vi "Load WAV.vi"(8 "error in (no error)":errorcluster, 11 "Path":path) -> (0 "error out":errorcluster, 1 "data":waveform(i16)[](array[waveform]), 2 "Sample Rate (Hz)":i32, 3 "Channels":i32, 5 "Length (Samples)":i32)   [LabVIEW 2018, in "Audio File Input.lvlib"]
doc: "Loads a WAV file from disk.\n\n<b>Priority:</b> Background priority (lowest)"
uses:
  Audio File Input.lvlib
  <vilib>/sound2/lvsound2.llb/Sound File Read Open.vi
  <vilib>/sound2/lvsound2.llb/Sound File Info (refnum).vi
  <vilib>/sound2/lvsound2.llb/Sound File Read (I16).vi
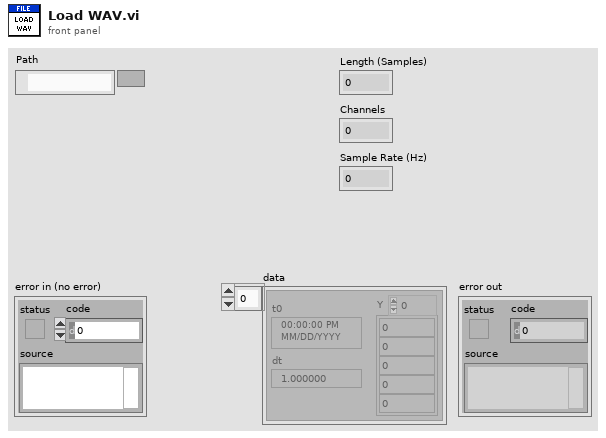
[diagram p1: front panel]
types:
  T1 = typedef "Sound File Refnum.ctl" = refnum<file>
  T2 = typedef "Sound Data Format.ctl" = cluster{"sample rate (S/s)":dbl, "number of channels":i32, "bits per sample":i32}
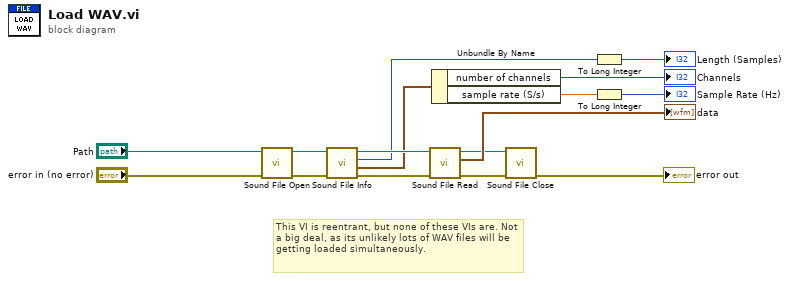
[diagram p0: block diagram]
diagram:
  # "This VI is reentrant, but none of these VIs are. Not a big deal, as its unlikely lots of WAV files will be getting loaded simultaneously."
  n1 = call-poly <vilib>:"Sound File Open.vi"("error in (no error)"="error in (no error)", "path"="Path") -> ("error out"=w8:errorcluster, "sound file refnum"=w9:T1)  [unwired: 8 in]
  n2 = call-poly <vilib>:"Sound File Info.vi"("error in (no error)"=w8, "sound file refnum"=w9) -> ("error out"=w6:errorcluster, "sound format"=w1:T2, "total number of samples/ch"=w3:u32, "sound file refnum out"=w7:T1)  [unwired: 6 in]
  n3 = call-poly <vilib>:"Sound File Read.vi"("error in (no error)"=w6, "sound file refnum"=w7) -> ("error out"=w4:errorcluster, "data"=→"data":waveform(i16)[], "sound file refnum out"=w5:T1)  [unwired: 5 in, 2 out]
  n4 = Unbundle By Name(w1) -> ("number of channels"=→"Channels":i32, "sample rate (S/s)"=w2:dbl)
  n5 = call <vilib>:"Sound File Close.vi"("error in (no error)"=w4, "sound file refnum"=w5) -> ("error out"=→"error out":errorcluster)  [unwired: 9 in]
  n6 = To Long Integer(number=w3) -> (32bit integer=→"Length (Samples)":i32)
  n7 = To Long Integer(number=w2) -> (32bit integer=→"Sample Rate (Hz)":i32)
